vi "Event Handler.vi"(0 "uService Template in":refnum<class "Waiter.lvclass">, 5 "Event type":T1=enum."Message", 7 "Item Name":string, 9 "Data":variant, 11 "error in (no error)":errorcluster) -> (4 "uService Template out":refnum<class "Waiter.lvclass">, 15 "error out":errorcluster)   [LabVIEW 2020, in "Waiter.lvlib" / "Waiter.lvclass"]
doc: "This VI is the event handler of the uService: every time an event is triggered to the uService, this VI is called.\nNote: here you can access the Actor/Class data, but it will be the one coming out from Init. You cannot modify the values.\nThree different events are supported:\nI) Button Pressed: get called on a GUI button pressed. Item Name is the name (label) of the button, Data is empty.\nII) Shared Variable Updated: get called when a SV you subscribed to is updated. Item Name is the name of the SV, and Data is the value (note: you need to convert it to the proper type).\nIII) Message: get called every time a user event is generated using Send Message to Event Handler. The values of Item Name and Data are the one given to the Send Message to Event Handler.\nIV) Ready to launch?: this frame get called every time a new Run is initiated. Each uService is responsible of performing a self check before giving back the green light for the Run to start."
uses:
  Waiter.lvclass
  Waiter.lvclass/Waiter.ctl
  TALOS/TALOS_PPL.lvlibp
  C:/LabVIEW Code/aegis-labview-code/TALOS/TALOS_PPL.lvlibp/Father of all uServices/Father of all uServices/Father of all uServices.lvclass
  C:/LabVIEW Code/aegis-labview-code/TALOS/TALOS_PPL.lvlibp/Ancestor/Ancestor/Ancestor.lvclass
  C:/LabVIEW Code/aegis-labview-code/TALOS/Actor Framework.lvlibp/1abvi3w/vi.lib/ActorFramework/Actor/Actor.lvclass
  TALOS/TALOS_PPL.lvlibp/Father of all uServices/Father of all uServices/Father of all uServices.lvclass
  WaiterConsumer Case Selector.ctl
  TALOS/TALOS_PPL.lvlibp/Father of all uServices/Father of all uServices/Event Handler Items.ctl
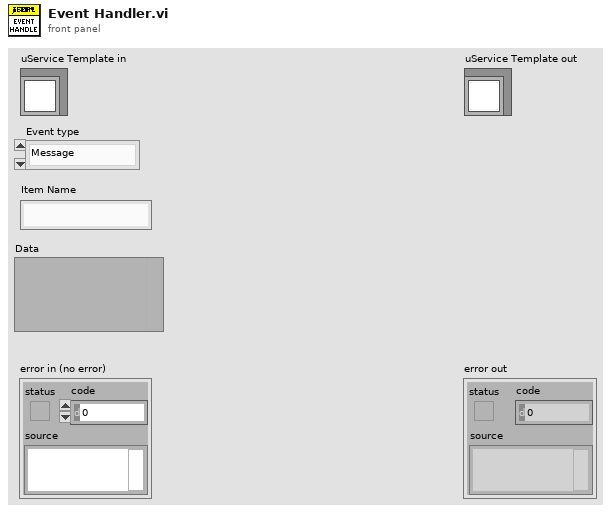
[diagram p1: front panel]
types:
  T1 = typedef "TALOS_PPL.lvlibp/Father of all uServices.lvlib/Father of all uServices.lvclass/Event Handler Items.ctl" = enum16{"Button Pressed", "Shared Variable Updated", "Message", "Ready to launch?", "Safe Mode", "Start RUN", "Stop RUN"}
  T2 = typedef "Waiter.lvlib/Waiter.lvclass/WaiterConsumer Case Selector.ctl" = enum16{"Send order to Pizza Machine"}
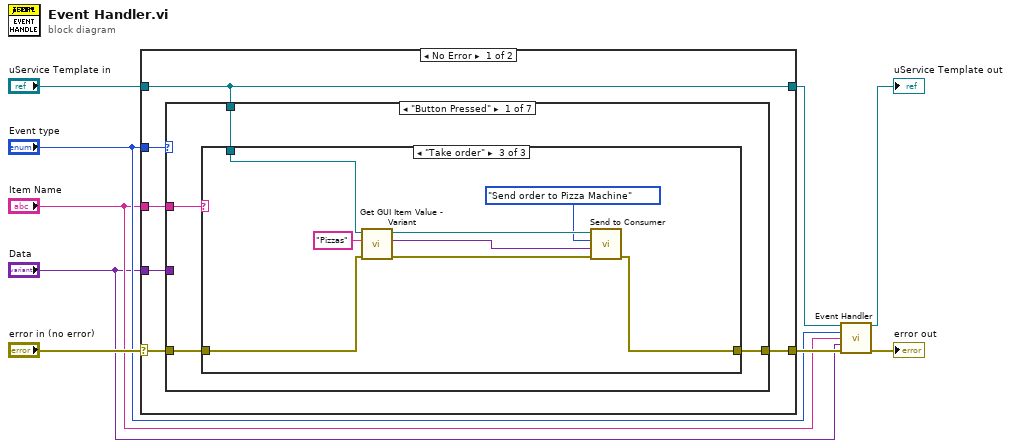
[diagram p0: block diagram]
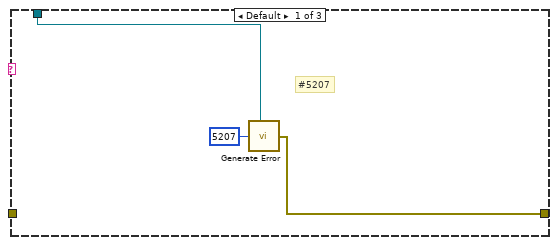
[diagram p2: hidden frame]
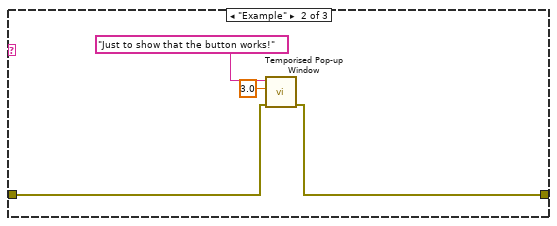
[diagram p3: hidden frame]
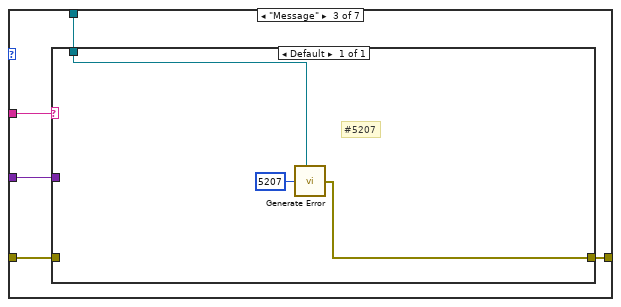
[diagram p5: hidden frame]
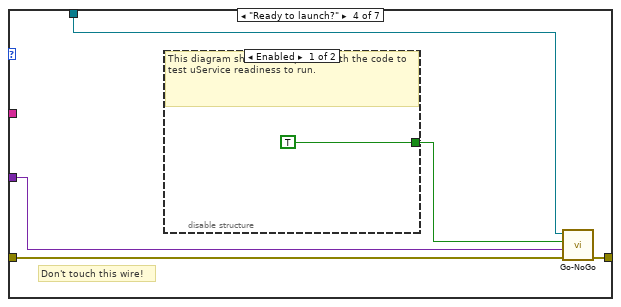
[diagram p6: hidden frame]
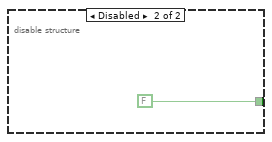
[diagram p7: hidden frame]
diagram:
  n1 = case shown="No Error" "error in (no error)" {
    selector: "error in (no error)" -> [w13 w55]
    tunnel: [w14 w55] -> w7
    tunnel: [w12 w54] -> w4
    tunnel: "uService Template in" -> [w12 w54]
    tunnel: "Event type" -> [w15 _]
    tunnel: "Item Name" -> [w11 _]
    tunnel: "Data" -> [w10 _]
    frame No Error {
      n2 = case shown="\"Button Pressed\"" w15 {
        tunnel: [w19 w35 w36 w47 w51 w52 w53] -> w14
        tunnel: w13 -> [w16 w35 w40 w48 w51 w52 w53]
        tunnel: w11 -> [w17 _ w39 _ _ _ _]
        tunnel: w12 -> [w18 _ w37 w46 _ _ _]
        tunnel: w10 -> [_ _ w38 w44 _ _ _]
        frame "Button Pressed" {
          n3 = case shown="\"Take order\"" w17 {
            tunnel: w16 -> [_ w23 w32]
            tunnel: [w20 w24 w30] -> w19
            tunnel: w18 -> [w21 _ w33]
            frame Default {
              # "#5207"
              n4 = call "Generate Error.vi"("Class"=w21, "Error Code"=5207) -> ("error out"=w20:errorcluster)  [unwired: 5 in]
            }
            frame "Example" {
              n5 = call "Temporised Pop-up Window.vi"("error in (no error)"=w23, "Timeout"=3.0, "Text"="Just to show that the button works!" ("message")) -> ("error out"=w24:errorcluster)  [unwired: 8 in]
            }
            frame "Take order" {
              n6 = call "Get GUI Item Value - Variant.vi"("error in (no error)"=w32, "FP Item Name"="Pizzas", "uService Template in"=w33) -> ("error out"=w31:errorcluster, "Value"=w27:variant, "uService Template out"=w29:refnum<class "Waiter.lvclass">)  [unwired: 6 in]
              n7 = call "Send to Consumer.vi"("error in (no error)"=w31, "Data"=w27, "Case ID"=WaiterConsumer_Case_Selector."Send order to Pizza Machine" ("Consumer Case Selector"), "uService Template in"=w29) -> ("error out"=w30:errorcluster)  [unwired: 6 in, 1 out]
            }
          }
        }
        frame "Shared Variable Updated" {
        }
        frame "Message" {
          n8 = case shown="Default" w39 {
            tunnel: w40 -> [_]
            tunnel: w38 -> [_]
            tunnel: w37 -> [w42]
            tunnel: [w41] -> w36
            frame Default {
              # "#5207"
              n9 = call "Generate Error.vi"("Class"=w42, "Error Code"=5207) -> ("error out"=w41:errorcluster)  [unwired: 5 in]
            }
          }
        }
        frame "Ready to launch?" {
          # "Don't touch this wire!"
          n10 = disable-structure shown="Enabled" {
            disable-tunnel: [TRUE ("Go?") FALSE ("Go?")] -> w45
            frame Enabled {
              # "This diagram should be replaced with the code to test uService readiness to run."
            }
            frame Disabled {
            }
          }
          n11 = call-dynamic "Go-NoGo.vi"("error in (no error)"=w48, "Go-NoGo Data"=w44, "Go?"=w45, "Father of all uServices in"=w46) -> ("error out"=w47:errorcluster)  [unwired: 6 in, 1 out]
        }
        frame "Safe Mode" {
          # "This case gets triggered"
        }
        frame "Start RUN" {
        }
        frame "Stop RUN" {
        }
      }
    }
    frame Error {
    }
  }
  n12 = call-parent "Event Handler.vi"("uService Template in"=w4, "Event type"="Event type", "Item Name"="Item Name", "Data"="Data", "error in (no error)"=w7) -> ("uService Template out"=→"uService Template out":refnum<class "Waiter.lvclass">, "error out"=→"error out":errorcluster)  [unwired: 9 in]
